vi "NEW NEW Tilt Platform Controller.vi"() -> ()   [LabVIEW 2014]
uses:
  <vilib>/Utility/file.llb/Read From Spreadsheet File (DBL).vi
  <vilib>/Utility/file.llb/Read From Spreadsheet File (I64).vi
  <vilib>/DAQmx/create/channels.llb/DAQmx Create Channel (DO-Digital Output).vi
  <vilib>/DAQmx/create/channels.llb/DAQmx Create Channel (AI-Voltage-Basic).vi
  <vilib>/DAQmx/configure/timing.llb/DAQmx Timing (Sample Clock).vi
  <vilib>/DAQmx/configure/trigger.llb/DAQmx Start Trigger (Digital Edge).vi
  <vilib>/DAQmx/create/channels.llb/DAQmx Create Channel (DI-Digital Input).vi
  <vilib>/DAQmx/read.llb/DAQmx Read (Analog 1D Wfm NChan NSamp).vi
  <vilib>/DAQmx/read.llb/DAQmx Read (Digital Bool 1Line 1Point).vi
  <vilib>/DAQmx/write.llb/DAQmx Write (Digital 1D Bool 1Chan 1Samp).vi
panel:
  out "Replay Loaded":bool
  in  "Parameter File":path
  in  "Load Sequence":bool
  in  "Replay File Path":path
  in  "Format":string="%.3f"
  in  "Delimiter":string=","
  in  "Column/Row Major":bool
  in  "Append to File?":bool=TRUE
  out "File Path":path
  out "Waveform Chart (Multiple Plots)":waveform(dbl)[](graph)
  in  "Callib Acce":bool
  in  "Callib Load Cell":bool
  in  "Transect?":bool
  in  "Week Number":dbl
  in  "Rat ID":string
  out "4/Ev8":bool
  out "5/Ev9":bool
  out "6/Ev10":bool
  out "2":bool
  out "1":bool
  out "3/Ev7":bool
  in  "Baseline Angle":dbl
  out "Angle":i32
  out "Total Force (g)":i32
  out "Completed Tilts":i32
  out "Current Tilt":i32
  out "Current ITI (s)":i32
  in  "Tirgger 6":bool=TRUE
  in  "Enable Left Slow":bool=TRUE
  in  "Enable Left Medium":bool=TRUE
  in  "Enable Left Fast":bool=TRUE
  in  "Enable Right Slow":bool=TRUE
  in  "Enable Right Medium":bool=TRUE
  in  "Enable Right Fast":bool=TRUE
  out "Left Slow":i32
  out "Left Medium":i32
  out "Left Fast":i32
  out "Right Slow":i32
  out "Right Medium":i32
  out "Right Fast":i32
  out "Practice?":bool
  in  "Stop 2":bool
  in  "Pause":bool=TRUE
  in  "Start":bool
  in  "Total Tilts":dbl=1000.0
  in  "ITI Base (s)":dbl=2.0 format="%#.2g"
  in  "ITI Random Multiplier":dbl=1.0 format="%#.2g"
  in  "Clock Source":i32(slide)=1 caption="Choose a setting:" scale=0.0..1.0
  out "Reward":bool
  # "Rat Ground Reaction Forces"
  # "Clock Source"
  # "Tilt Parameters"
  # "Animal Info"
  # "Right"
  # "Left"
  # "Current Values"
  # "Enable"
  # "Enable"
  # "Callibration"
  # "File Information"
  # "Replay Sequence"
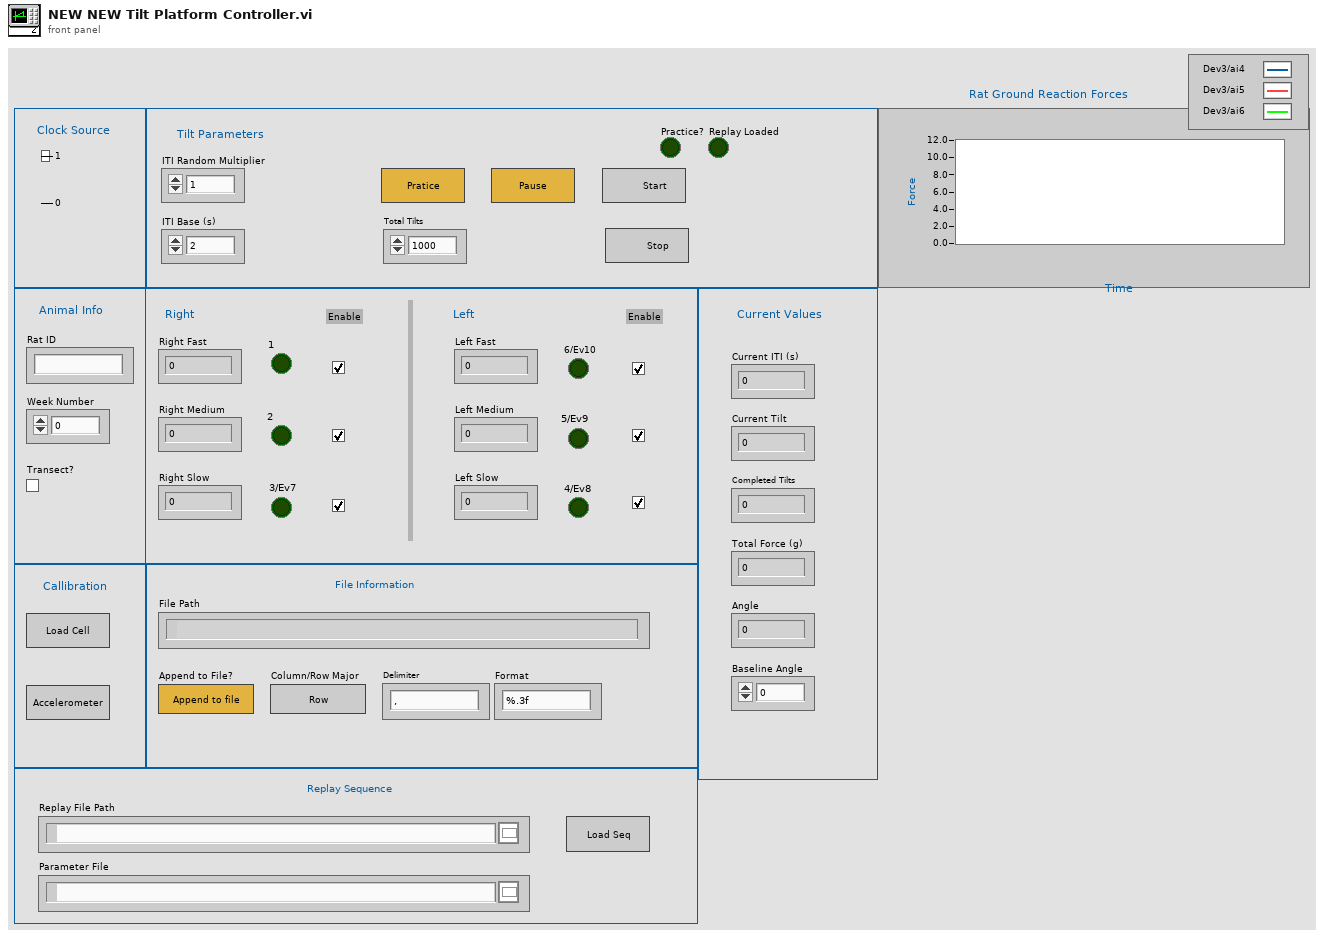
[diagram p1: front panel]
types:
  T1 = enum16{"open", "replace", "create", "open or create", "replace or create", "replace or create with confirmation"}
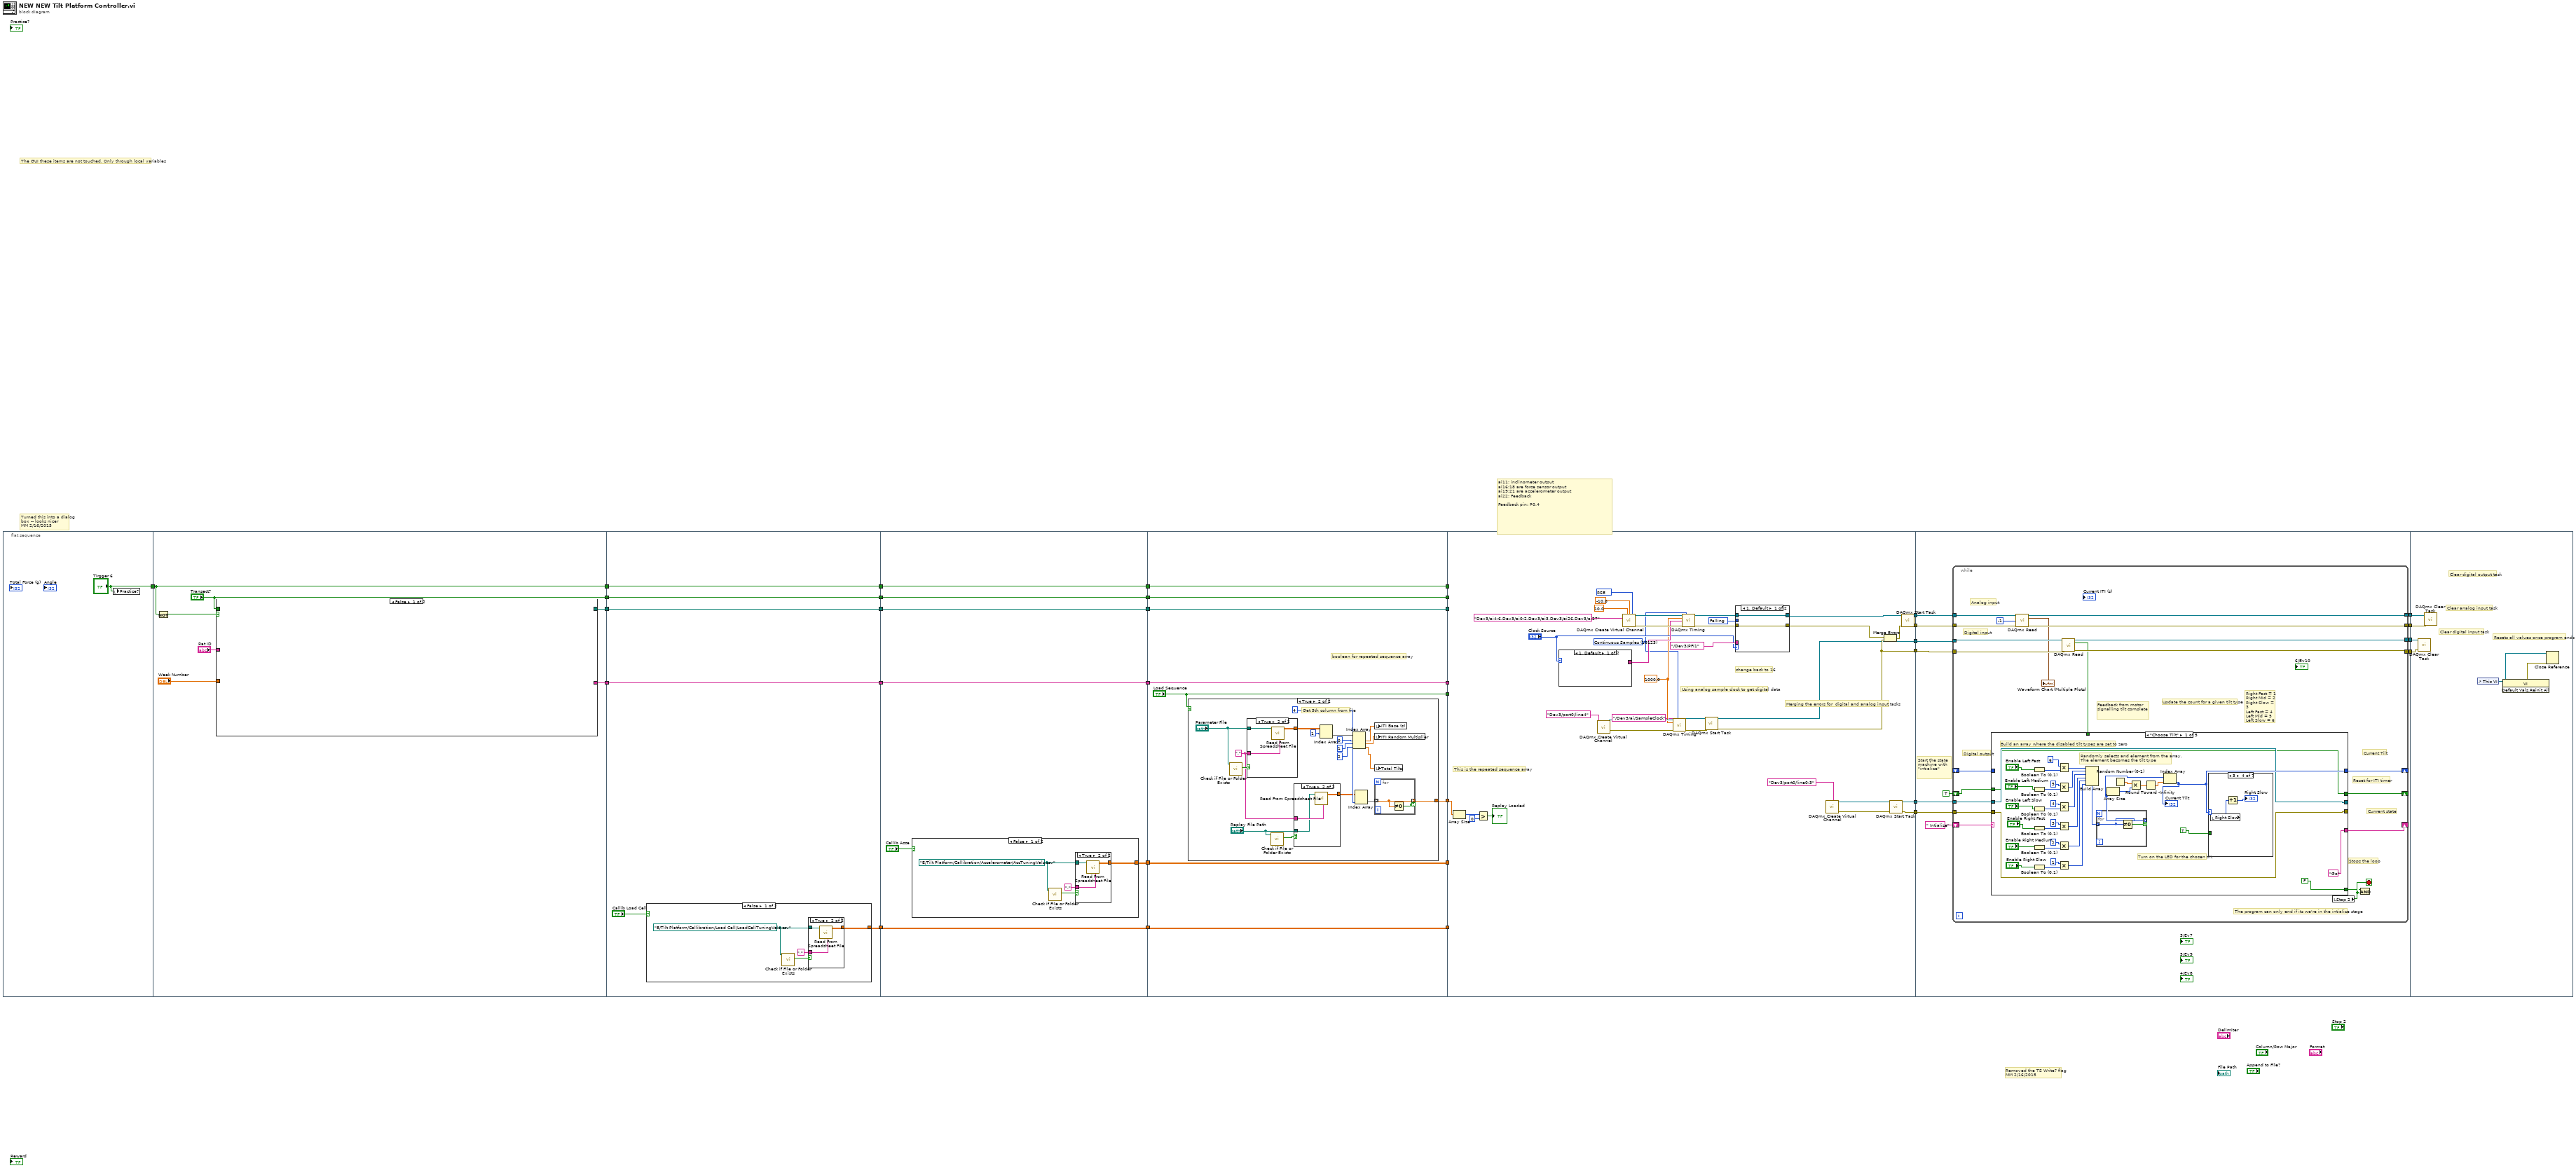
[diagram p0: block diagram]
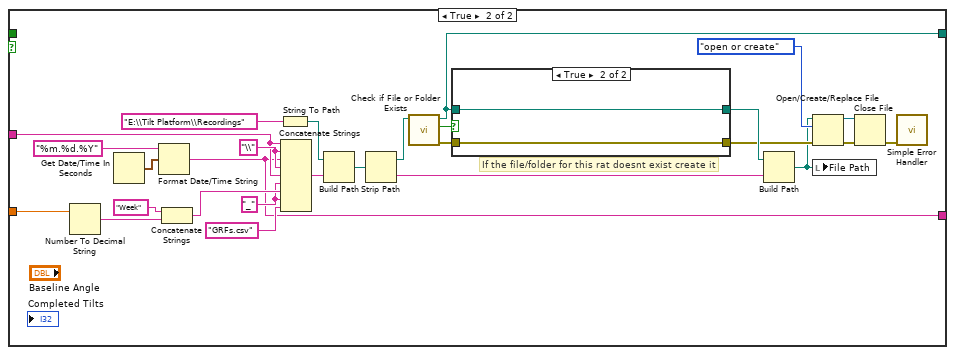
[diagram p2: hidden frame]
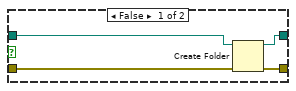
[diagram p3: hidden frame]
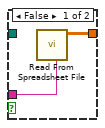
[diagram p4: hidden frame]
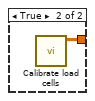
[diagram p5: hidden frame]
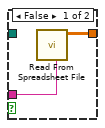
[diagram p6: hidden frame]
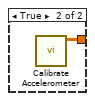
[diagram p7: hidden frame]
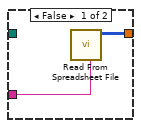
[diagram p9: hidden frame]
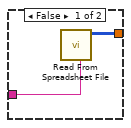
[diagram p10: hidden frame]
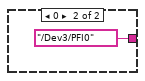
[diagram p11: hidden frame]
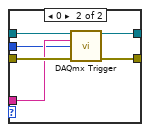
[diagram p12: hidden frame]
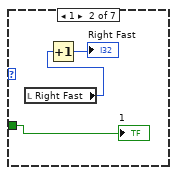
[diagram p14: hidden frame]
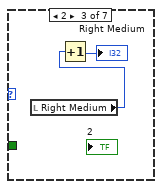
[diagram p15: hidden frame]
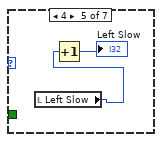
[diagram p16: hidden frame]
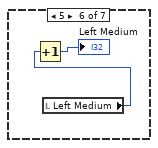
[diagram p17: hidden frame]
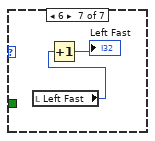
[diagram p18: hidden frame]
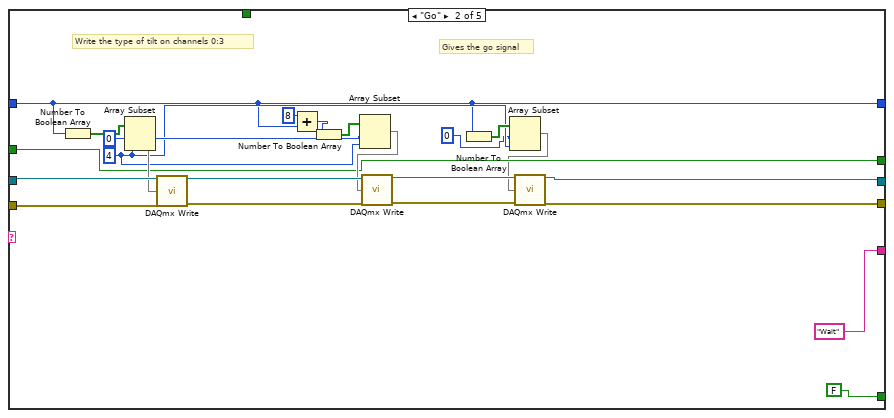
[diagram p19: hidden frame]
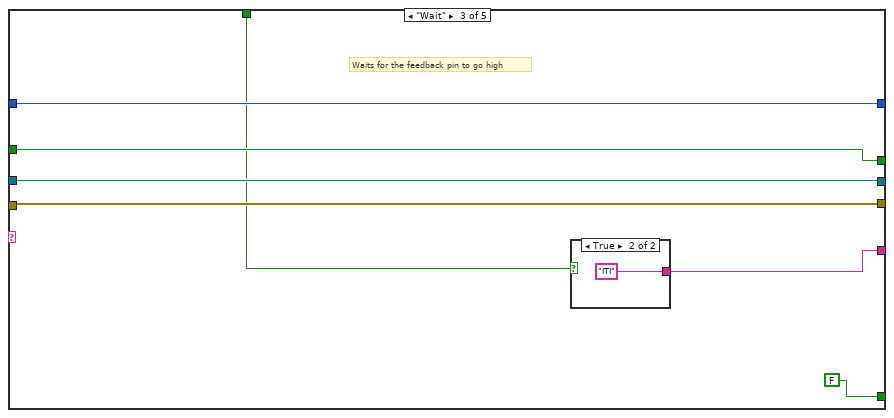
[diagram p20: hidden frame]
diagram:
  # "Removed the TS Write? flag\nMM 2/16/2015"
  # "ai11: inclinometer output \nai16:18 are force sensor output\nai19:21 are accelerometer output\nai22: Feedback\n\nFeedback pin: P0.4"
  # "Turned this into a dialog\nbox -- looks nicer\nMM 2/16/2015"
  # "The GUI these items are not touched. Only through local variables"
  n1 = flat-sequence {
    tunnel: ["Tirgger 6"] -> w34
    tunnel: w34 -> [w39]
    tunnel: [w39] -> w33
    tunnel: [w42] -> w32
    tunnel: ["Transect?"] -> w24
    tunnel: [w36] -> w23
    tunnel: w33 -> [w81]
    tunnel: [w81] -> w31
    tunnel: w32 -> [w79]
    tunnel: [w80] -> w30
    tunnel: [w79] -> w29
    tunnel: [w77] -> w25
    tunnel: w24 -> [w77]
    tunnel: w23 -> [w76]
    tunnel: [w76] -> w22
    tunnel: [w98] -> w21
    tunnel: w31 -> [w97]
    tunnel: [w97] -> w19
    tunnel: w30 -> [w98]
    tunnel: [w96] -> w17
    tunnel: [w95] -> w15
    tunnel: w29 -> [w95]
    tunnel: w25 -> [w93]
    tunnel: [w93] -> w13
    tunnel: [w92] -> w11
    tunnel: w22 -> [w92]
    tunnel: w21 -> [w116]
    tunnel: [w116] -> w20
    tunnel: w19 -> [w115]
    tunnel: [w115] -> w18
    tunnel: w17 -> [w114]
    tunnel: [w114] -> w16
    tunnel: w15 -> [w113]
    tunnel: [w113] -> w14
    tunnel: w13 -> [w112]
    tunnel: [w112] -> w12
    tunnel: w11 -> [w111]
    tunnel: [w111] -> w10
    tunnel: ["Load Sequence"] -> w9
    tunnel: [w109] -> w8
    tunnel: [w179] -> w28
    tunnel: w20 -> [_]
    tunnel: w18 -> [_]
    tunnel: [w169] -> w27
    tunnel: [w168] -> w26
    tunnel: w16 -> [_]
    tunnel: w14 -> [_]
    tunnel: w12 -> [_]
    tunnel: w10 -> [_]
    tunnel: w9 -> [_]
    tunnel: w8 -> [w166]
    tunnel: [w155] -> w7
    tunnel: [w154] -> w6
    tunnel: [w147] -> w1
    tunnel: w28 -> [w201]
    tunnel: w27 -> [w200]
    tunnel: w26 -> [w198]
    tunnel: w7 -> [w203]
    tunnel: w6 -> [w202]
    tunnel: [w199] -> w5
    tunnel: [w197] -> w4
    tunnel: [w196] -> w3
    tunnel: [w195] -> w2
    tunnel: w1 -> [w193]
    tunnel: w5 -> [w355]
    tunnel: w4 -> [w354]
    tunnel: w3 -> [w353]
    tunnel: w2 -> [w352]
    frame #0 {
      n2 = local write "Practice?"("Tirgger 6") -> ()
    }
    frame #1 {
      n3 = Not(x=w39) -> (.not. x?=w38:bool)
      n4 = case shown="False" w38 {
        tunnel: "Transect?" -> [_ _]
        tunnel: "Week Number" -> [_ w47]
        tunnel: "Rat ID" -> [_ w46]
        tunnel: [_ w45] -> w42
        tunnel: [_ w43] -> w36
        frame False {
        }
        frame True {
          w48 = "_"
          w53 = "\\" ("string")
          # "If the file/folder for this rat doesnt exist create it"
          n5 = Number To Decimal String(number=w47) -> (decimal integer string=w68:string)  [unwired: 1 in]
          n6 = Get Date/Time In Seconds() -> (seconds since 1Jan1904=w65:timestamp)
          n7 = Format Date/Time String(time format string (%c)="%m.%d.%Y", seconds (now)=w65) -> (date/time string=w43:string)  [unwired: 1 in]
          n8 = Concatenate Strings("Week" ("string"), w68) -> (w52:string)
          n9 = String To Path(string="E:\\Tilt Platform\\Recordings") -> (path=w67:path)
          n10 = Concatenate Strings(w46, w53, w43, w53, w46, w48, w52, w48, "GRFs.csv" ("string")) -> (w50:string)
          n11 = Build Path(base path=w67, name or relative path=w50) -> (appended path=w63:path)
          n12 = Strip Path(path=w63) -> (stripped path=w62:path, name=w51:string)
          n13 = call <vilib>:"Check if File or Folder Exists.vi"("path"=w62) -> ("error out"=w60:errorcluster, "file or folder exists?"=w61:bool, "dup path"=w45:path)  [unwired: 8 in]
          n14 = case shown="True" w61 {
            tunnel: w45 -> [w73 w75]
            tunnel: w60 -> [w72 w74]
            tunnel: [w71 w75] -> w57
            tunnel: [w70 w74] -> w56
            frame False {
              n15 = Create Folder(path (use dialog)=w73, error in=w72) -> (created path=w71:path, error out=w70:errorcluster)  [unwired: 1 in, 1 out]
            }
            frame True {
            }
          }
          n16 = Build Path(base path=w57, name or relative path=w51) -> (appended path=w44:path)
          n17 = Open/Create/Replace File(file path (use dialog)=w44, error in=w56, operation (0:open)=T1."open or create") -> (refnum out=w59:refnum<file>, error out=w55:errorcluster)  [unwired: 3 in, 1 out]
          n18 = local write "File Path"(w44) -> ()
          n19 = Close File(refnum=w59, error in=w55) -> (error out=w54:errorcluster)  [unwired: 1 out]
          n20 = call <vilib>:"Simple Error Handler.vi"("error in (no error)"=w54) -> ()  [unwired: 4 in, 5 out]
        }
      }
    }
    frame #2 {
      n21 = case shown="False" "Callib Load Cell" {
        tunnel: [w83 w91] -> w80
        frame False {
          w84 = path "E:/Tilt Platform/Callibration/Load Cell/LoadCellTuningVals.csv" ("file path (dialog if empty)")
          n22 = call <vilib>:"Check if File or Folder Exists.vi"("path"=w84) -> ("file or folder exists?"=w85:bool)  [unwired: 8 in, 2 out]
          n23 = case shown="True" w85 {
            tunnel: w84 -> [_ w90]
            tunnel: [w87 w89] -> w83
            tunnel: "," ("delimiter (\\t)") -> [w86 w88]
            frame False {
              n24 = call-poly <vilib>:"Read From Spreadsheet File.vi"("delimiter (\\t)"=w86) -> ("all rows"=w87:dbl[][])  [unwired: 6 in, 4 out]
            }
            frame True {
              n25 = call-poly <vilib>:"Read From Spreadsheet File.vi"("delimiter (\\t)"=w88, "file path (dialog if empty)"=w90) -> ("all rows"=w89:dbl[][])  [unwired: 5 in, 4 out]
            }
          }
        }
        frame True {
          n26 = call "Calibrate load cells.vi"() -> ("Slope and Intercept"=w91:dbl[][])  [unwired: 11 in]
        }
      }
    }
    frame #3 {
      n27 = case shown="False" "Callib Acce" {
        tunnel: [w101 w108] -> w96
        frame False {
          w100 = path "E:/Tilt Platform/Callibration/Accelerometer/AccTuningVals.csv" ("file path (dialog if empty)")
          n28 = call <vilib>:"Check if File or Folder Exists.vi"("path"=w100) -> ("file or folder exists?"=w99:bool)  [unwired: 8 in, 2 out]
          n29 = case shown="True" w99 {
            tunnel: "," ("delimiter (\\t)") -> [w103 w107]
            tunnel: [w104 w106] -> w101
            tunnel: w100 -> [_ w105]
            frame False {
              n30 = call-poly <vilib>:"Read From Spreadsheet File.vi"("delimiter (\\t)"=w103) -> ("all rows"=w104:dbl[][])  [unwired: 6 in, 4 out]
            }
            frame True {
              n31 = call-poly <vilib>:"Read From Spreadsheet File.vi"("delimiter (\\t)"=w107, "file path (dialog if empty)"=w105) -> ("all rows"=w106:dbl[][])  [unwired: 5 in, 4 out]
            }
          }
        }
        frame True {
          n32 = call "Calibrate Accelerometer.vi"() -> ("Output"=w108:dbl[][])  [unwired: 9 in]
        }
      }
    }
    frame #4 {
      # "boolean for repeated sequence array"
      n33 = case shown="True" "Load Sequence" {
        tunnel: [_ w130] -> w109
        frame False {
        }
        frame True {
          w126 = "," ("delimiter (\\t)")
          # "Get 5th column from file"
          n34 = call <vilib>:"Check if File or Folder Exists.vi"("path"="Parameter File") -> ("file or folder exists?"=w128:bool)  [unwired: 8 in, 2 out]
          n35 = case shown="True" w128 {
            tunnel: w126 -> [w136 w139]
            tunnel: "Parameter File" -> [_ w138]
            tunnel: [w135 w137] -> w125
            frame False {
              n36 = call-poly <vilib>:"Read From Spreadsheet File.vi"("delimiter (\\t)"=w136) -> ("all rows"=w135:i64[][])  [unwired: 6 in, 4 out]
            }
            frame True {
              n37 = call-poly <vilib>:"Read From Spreadsheet File.vi"("delimiter (\\t)"=w139, "file path (dialog if empty)"=w138) -> ("all rows"=w137:dbl[][])  [unwired: 5 in, 4 out]
            }
          }
          n38 = call <vilib>:"Check if File or Folder Exists.vi"("path"="Replay File Path") -> ("file or folder exists?"=w134:bool)  [unwired: 8 in, 2 out]
          n39 = case shown="True" w134 {
            tunnel: w126 -> [w143 w146]
            tunnel: "Replay File Path" -> [_ w145]
            tunnel: [w142 w144] -> w131
            frame False {
              n40 = call-poly <vilib>:"Read From Spreadsheet File.vi"("delimiter (\\t)"=w143) -> ("all rows"=w142:i64[][])  [unwired: 6 in, 4 out]
            }
            frame True {
              n41 = call-poly <vilib>:"Read From Spreadsheet File.vi"("delimiter (\\t)"=w146, "file path (dialog if empty)"=w145) -> ("all rows"=w144:dbl[][])  [unwired: 5 in, 4 out]
            }
          }
          n42 = Index Array(array=w125, index (row)=1) -> (element=w123:dbl[])  [unwired: 1 in]
          n43 = Index Array(array=w123, index #1=0 ("index"), index #2=1 ("index"), index #3=2 ("index")) -> (element #1=w119:dbl, element #2=w118:dbl, element #3=w117:dbl)
          n44 = Index Array(array=w131, index (col)=4 ("index")) -> (element=w129:dbl[])  [unwired: 1 in]
          n45 = local write "ITI Base (s)"(w119) -> ()
          n46 = local write "ITI Random Multiplier"(w118) -> ()
          n47 = local write "Total Tilts"(w117) -> ()
          n48 = for {
            tunnel: [w141] -> w130 mode=indexing if=w140
            tunnel: w129 -> [w141] mode=indexing
            n49 = Not Equal To 0?(x=w141) -> (x != 0?=w140:bool)
          }
        }
      }
    }
    frame #5 {
      w170 = 10171 items=["Rising"=10280, "Falling"=10171] ("edge")
      w152 = 10123 items=["Finite Samples"=10178, "Continuous Samples"=10123, "Hardware Timed Single Point"=12522] ("sample mode")
      w173 = 10083 items=["default"=-1, "RSE"=10083, "NRSE"=10078, "Differential"=10106, "Pseudodifferential"=12529] ("input terminal configuration")
      w159 = 1000.0 ("rate")
      # "Merging the errors for  digital and analog input tasks"
      # "Using analog sample clock to get digital data"
      # "change back to 16"
      # "This is the repeated sequence array"
      n50 = Array Size(array=w166) -> (size(s)=w165:i32)
      n51 = Greater?(x=w165, y=0) -> (0:→"Replay Loaded":bool)
      n52 = case shown="1, Default" "Clock Source" {
        tunnel: [_ tag "/Dev3/PFI0" ("source")] -> w172
        frame 1, Default {
        }
        frame 0 {
        }
      }
      n53 = call-poly <vilib>:"DAQmx Create Virtual Channel.vi"("lines"=tag "Dev3/port0/line4") -> ("task out"=w160:refnum<k21>, "error out"=w161:errorcluster)  [unwired: 13 in]
      n54 = call-poly <vilib>:"DAQmx Create Virtual Channel.vi"("maximum value"=10.0, "minimum value"=-10.0, "input terminal configuration"=w173, "physical channels"=tag "Dev3/ai4:6,Dev3/ai0:2,Dev3/ai3,Dev3/ai26,Dev3/ai27") -> ("task out"=w174:refnum<k21>, "error out"=w175:errorcluster)  [unwired: 10 in]
      n55 = call-poly <vilib>:"DAQmx Timing.vi"("task/channels in"=w160, "sample mode"=w152, "rate"=w159, "source"=tag "/Dev3/ai/SampleClock", "error in"=w161) -> ("task out"=w157:refnum<k21>, "error out"=w156:errorcluster)  [unwired: 9 in]
      n56 = call-poly <vilib>:"DAQmx Timing.vi"("task/channels in"=w174, "sample mode"=w152, "rate"=w159, "source"=w172, "error in"=w175) -> ("task out"=w150:refnum<k21>, "error out"=w151:errorcluster)  [unwired: 9 in]
      n57 = call <vilib>:"DAQmx Start Task.vi"("task/channels in"=w157, "error in"=w156) -> ("task out"=w154:refnum<k21>, "error out"=w155:errorcluster)  [unwired: 12 in]
      n58 = case shown="1, Default" "Clock Source" {
        tunnel: w150 -> [w185 w191]
        tunnel: w151 -> [w184 w190]
        tunnel: tag "/Dev3/PFI1" ("source") -> [_ w189]
        tunnel: w170 -> [_ w188]
        tunnel: [w185 w186] -> w149
        tunnel: [w184 w187] -> w148
        frame 1, Default {
        }
        frame 0 {
          n59 = call-poly <vilib>:"DAQmx Trigger.vi"("task/channels in"=w191, "source"=w189, "edge"=w188, "error in"=w190) -> ("task out"=w186:refnum<k21>, "error out"=w187:errorcluster)  [unwired: 10 in]
        }
      }
      n60 = call-poly <vilib>:"DAQmx Create Virtual Channel.vi"("lines"=tag "Dev3/port0/line0:3") -> ("task out"=w181:refnum<k21>, "error out"=w180:errorcluster)  [unwired: 13 in]
      n61 = Merge Errors(w148, w155) -> (w153:errorcluster)
      n62 = call <vilib>:"DAQmx Start Task.vi"("task/channels in"=w181, "error in"=w180) -> ("task out"=w179:refnum<k21>, "error out"=w147:errorcluster)  [unwired: 12 in]
      n63 = call <vilib>:"DAQmx Start Task.vi"("task/channels in"=w149, "error in"=w153) -> ("task out"=w169:refnum<k21>, "error out"=w168:errorcluster)  [unwired: 12 in]
    }
    frame #6 {
      # "Start the state machine with \"intialize\""
      n64 = while {
        tunnel: w203 -> [w218]
        tunnel: w202 -> [w223]
        tunnel: w201 -> [w212]
        tunnel: w193 -> [w211]
        tunnel: [w222] -> w199
        tunnel: w200 -> [w224]
        tunnel: w198 -> [w221]
        tunnel: [w220] -> w197
        tunnel: [w219] -> w196
        tunnel: [w217] -> w195
        shift-right: [w214] -> _
        shift-left: " Intialize" -> [w215]
        shift-right: [w210] -> _
        shift-left: _ -> [w209]
        shift-right: [w207] -> _
        shift-left: TRUE ("Time has Elapsed") -> [w206]
        stop <- w205 stop-if-true
        # "The program can only end if its we're in the intialize stage"
        # "Currrent state"
        # "Reset for ITI timer"
        # "Feedback from motor signalling tilt complete"
        # "Current Tilt"
        # "Update the count for a given tilt type"
        # "Right Fast = 1\nRight Mid = 2\nRight Slow = 3\nLeft Fast = 4\nLeft Mid = 5\nLeft Slow = 6"
        # "Stops the loop"
        # "Digital input"
        # "Analog input"
        # "Digital output"
        n65 = call-poly <vilib>:"DAQmx Read.vi"("task/channels in"=w224, "number of samples per channel"=-1, "error in"=w221) -> ("task out"=w222:refnum<k21>, "data"=→"Waveform Chart (Multiple Plots)":waveform(dbl)[], "error out"=w220:errorcluster)  [unwired: 10 in]
        n66 = call-poly <vilib>:"DAQmx Read.vi"("task/channels in"=w223, "error in"=w218) -> ("task out"=w219:refnum<k21>, "data"=w208:bool, "error out"=w217:errorcluster)  [unwired: 11 in]
        n67 = case shown="\"Choose Tilt\"" w215 {
          tunnel: ["Go" "Wait" w304 w312 w348] -> w214
          tunnel: w212 -> [w229 w298 w306 w315 w346]
          tunnel: w211 -> [w228 w297 w305 w314 w345]
          tunnel: [w230 w278 w303 w316 w347] -> w210
          tunnel: w209 -> [_ w278 w303 w316 w347]
          tunnel: [w229 w286 w306 w315 w346] -> _
          tunnel: [w228 w285 w305 w314 w345] -> _
          tunnel: w208 -> [_ _ w301 _ _]
          tunnel: [w227 w289 w302 w313 w344] -> w207
          tunnel: w206 -> [w227 w289 w302 w311 w344]
          tunnel: [FALSE FALSE FALSE FALSE TRUE] -> w204
          frame "Choose Tilt" {
            # "Turn on the LED for the chosen tilt"
            # "Randomly selects and element from the array.\nThe element becomes the tilt type"
            # "Build an array where the disabled tilt types are set to zero"
            n68 = Boolean To (0,1)(Boolean="Enable Left Fast") -> (0, 1=w255:i16)
            n69 = Boolean To (0,1)(Boolean="Enable Left Medium") -> (0, 1=w254:i16)
            n70 = Boolean To (0,1)(Boolean="Enable Left Slow") -> (0, 1=w253:i16)
            n71 = Boolean To (0,1)(Boolean="Enable Right Fast") -> (0, 1=w252:i16)
            n72 = Boolean To (0,1)(Boolean="Enable Right Medium") -> (0, 1=w251:i16)
            n73 = Boolean To (0,1)(Boolean="Enable Right Slow") -> (0, 1=w250:i16)
            n74 = Multiply(x=6, y=w255) -> (x*y=w249:i32)
            n75 = Multiply(x=5, y=w254) -> (x*y=w248:i32)
            n76 = Multiply(x=4, y=w253) -> (x*y=w247:i32)
            n77 = Multiply(x=3, y=w252) -> (x*y=w246:i32)
            n78 = Multiply(x=2, y=w251) -> (x*y=w245:i32)
            n79 = Multiply(x=1, y=w250) -> (x*y=w244:i32)
            n80 = Build Array(w249, w248, w247, w246, w245, w244) -> (w243:i32[])
            n81 = for {
              tunnel: [w275] -> w232 mode=indexing if=w276
              tunnel: w243 -> [w275] mode=indexing
              n82 = Not Equal To 0?(x=w275) -> (x != 0?=w276:bool)
            }
            n83 = Array Size(array=w232) -> (size(s)=w234:i32)
            n84 = Random Number (0-1)() -> (number: 0 to 1=w236:dbl)
            n85 = Multiply(x=w236, y=w234) -> (x*y=w235:dbl)
            n86 = Round Toward -Infinity(1:w235) -> (0:w233:dbl)
            n87 = Index Array(array=w232, index=w233) -> (element=w230:i32)
            "Current Tilt" <- w230
            n88 = case shown="3" w230 {
              tunnel: TRUE -> [_ w262 _ _ _ _ _]
              frame Default {
              }
              frame 1 {
                n89 = local read "Right Fast"() -> (w263:i32)
                n90 = Increment(x=w263) -> (x+1=→"Right Fast":i32)
                "1" <- w262
              }
              frame 2 {
                n91 = local read "Right Medium"() -> (w265:i32)
                n92 = Increment(x=w265) -> (x+1=→"Right Medium":i32)
              }
              frame 3 {
                n93 = local read "Right Slow"() -> (w267:i32)
                n94 = Increment(x=w267) -> (x+1=→"Right Slow":i32)
              }
              frame 4 {
                n95 = local read "Left Slow"() -> (w269:i32)
                n96 = Increment(x=w269) -> (x+1=→"Left Slow":i32)
              }
              frame 5 {
                n97 = local read "Left Medium"() -> (w271:i32)
                n98 = Increment(x=w271) -> (x+1=→"Left Medium":i32)
              }
              frame 6 {
                n99 = local read "Left Fast"() -> (w273:i32)
                n100 = Increment(x=w273) -> (x+1=→"Left Fast":i32)
              }
            }
          }
          frame "Go" {
            w282 = 4 ("length")
            w291 = 0 ("index")
            # "Gives the go signal"
            # "Write the type of tilt on channels 0:3"
            n101 = Number To Boolean Array(number=w278) -> (Boolean array=w294:bool[])
            n102 = Array Subset(array=w294, index=w291, length=w282) -> (w293:bool[])
            n103 = call-poly <vilib>:"DAQmx Write.vi"("task/channels in"=w298, "data"=w293, "error in"=w297) -> ("task out"=w296:refnum<k21>, "error out"=w295:errorcluster)  [unwired: 10 in, 1 out]
            n104 = Add(x=u8 8, y=w278) -> (x+y=w280:i32)
            n105 = Number To Boolean Array(number=w280) -> (Boolean array=w292:bool[])
            n106 = Array Subset(array=w292, index=w291, length=w282) -> (w290:bool[])
            n107 = call-poly <vilib>:"DAQmx Write.vi"("task/channels in"=w296, "data"=w290, "error in"=w295) -> ("task out"=w288:refnum<k21>, "error out"=w287:errorcluster)  [unwired: 10 in, 1 out]
            n108 = Number To Boolean Array(number=w278) -> (Boolean array=w284:bool[])
            n109 = Array Subset(array=w284, index=u8 0, length=w282) -> (w283:bool[])
            n110 = call-poly <vilib>:"DAQmx Write.vi"("task/channels in"=w288, "data"=w283, "error in"=w287) -> ("task out"=w286:refnum<k21>, "error out"=w285:errorcluster)  [unwired: 10 in, 1 out]
          }
          frame "Wait" {
            # "Waits for the feedback pin to go high"
            n111 = case shown="True" w301 {
              tunnel: ["Wait" "ITI"] -> w304
              frame False {
              }
              frame True {
              }
            }
          }
          frame "ITI" {
            # "Checks that the designated time has elapsed"
            # "Chooses a random inter trial interval. After the initial randomization it doesn't randomize again."
            n112 = call "Elapsed Time"("Time Target (s)"="ITI Base (s)", "Reset"=w311, "Auto Reset"=FALSE) -> ("Time has Elapsed"=w313:bool)  [unwired: 9 in, 7 out]
            n113 = case shown="False" w313 {
              tunnel: ["ITI" "Intialize"] -> w312
              frame False {
              }
              frame True {
              }
            }
          }
          frame "Intialize", Default {
            w349 = FALSE
            n114 = local read "Left Medium"() -> (w332:i32)
            n115 = local read "Left Slow"() -> (w326:i32)
            n116 = local read "Right Fast"() -> (w338:i32)
            n117 = local read "Right Medium"() -> (w335:i32)
            n118 = local read "Left Fast"() -> (w333:i32)
            n119 = local read "Right Slow"() -> (w334:i32)
            n120 = local write "6/Ev10"(w349) -> ()
            n121 = local write "3/Ev7"(w349) -> ()
            n122 = local write "4/Ev8"(w349) -> ()
            n123 = local write "5/Ev9"(w349) -> ()
            n124 = local write "1"(w349) -> ()
            n125 = local write "2"(w349) -> ()
            n126 = Greater Or Equal?(x=w338, y="Total Tilts") -> (x >= y?=w337:bool)
            n127 = Greater Or Equal?(x=w335, y="Total Tilts") -> (x >= y?=w331:bool)
            n128 = Greater Or Equal?(x=w333, y="Total Tilts") -> (x >= y?=w329:bool)
            n129 = Greater Or Equal?(x=w334, y="Total Tilts") -> (x >= y?=w330:bool)
            n130 = Greater Or Equal?(x=w332, y="Total Tilts") -> (x >= y?=w328:bool)
            n131 = Greater Or Equal?(x=w326, y="Total Tilts") -> (x >= y?=w327:bool)
            n132 = Not(x=w337) -> (.not. x?=w336:bool)
            n133 = Not(x=w331) -> (.not. x?=w325:bool)
            n134 = Not(x=w327) -> (.not. x?=w321:bool)
            n135 = Not(x=w328) -> (.not. x?=w322:bool)
            n136 = Not(x=w330) -> (.not. x?=w324:bool)
            n137 = Not(x=w329) -> (.not. x?=w323:bool)
            n138 = local write "Enable Right Slow"(w324) -> ()
            n139 = local write "Enable Left Fast"(w323) -> ()
            n140 = local write "Enable Right Medium"(w325) -> ()
            n141 = local write "Enable Left Slow"(w321) -> ()
            n142 = local write "Enable Right Fast"(w336) -> ()
            n143 = local write "Enable Left Medium"(w322) -> ()
            n144 = Not(x="Pause") -> (.not. x?=w342:bool)
            n145 = And(x="Start", y=w342) -> (x .and. y?=w340:bool)
            n146 = case shown="False" w340 {
              tunnel: ["Intialize" "Choose Tilt"] -> w348
              frame False {
              }
              frame True {
              }
            }
          }
        }
        n147 = local read "Stop 2"() -> (w205:bool)
        n148 = And(x=w204, y=w205) -> ()  [unwired: 1 out]
      }
    }
    frame #7 {
      # "Clear digital input task"
      # "Clear analog input task"
      # "Clear digital output task"
      # "Resets all values once program ends"
      n149 = call <vilib>:"DAQmx Clear Task.vi"("task in"=w353, "error in"=w352) -> ()  [unwired: 13 in, 1 out]
      n150 = call <vilib>:"DAQmx Clear Task.vi"("task in"=w355, "error in"=w354) -> ()  [unwired: 13 in, 1 out]
      n151 = control-ref of="This VI"() -> (w358:refnum<vi>)
      n152 = invoke class="VI" method="Default Vals.Reinit All"(reference=w358) -> (reference out=w356:refnum<vi>, error out=w357:errorcluster)  [unwired: 2 in, 1 out]
      n153 = Close Reference(reference=w356, error in (no error)=w357) -> ()  [unwired: 1 out]
    }
  }
